vi "Configure Channels.vi"(8 "error in":errorcluster, 11 "AI Voltage DAQmx Cont CFG in":refnum<class "AI Voltage DAQmx Cont CFG.lvclass">) -> (0 "error out":errorcluster, 3 "AI Voltage DAQmx Cont CFG out":refnum<class "AI Voltage DAQmx Cont CFG.lvclass">)   [LabVIEW 2023, in "AI Voltage DAQmx Cont CFG.lvclass"]
uses:
  AI Voltage DAQmx Cont CFG.lvclass
  AI Voltage DAQmx Cont CFG.lvclass/AI Voltage DAQmx Cont CFG.ctl
  <vilib>/Utility/error.llb/Error Cluster From Error Code.vi
  <vilib>/ErrorRing/Error Ring.xnode
  Configuration/Configuration JSON/Configuration JSON Base/CFG JSON.lvclass
  809d0f84-c2e6-4280-b3a5-eb032ce861ff.vi
  DAQmx/DAQmx Base CFG/DAQmx Base CFG.lvclass
  D:/git/HAL/HAL GOOP4/DAQmx/DAQmx BufferLastReadsDBL/DAQmx BufferLastReadsDBL.lvclass
  D:/git/HAL/HAL GOOP4/DAQmx/DAQmx Base CFG/DAQmx Base CFG.lvclass
  D:/git/HAL/HAL GOOP4/CFG Target/CFG Target.lvclass
  D:/git/HAL/HAL GOOP4/Configuration/Configuration Semaphore/CFG Semaphore.lvclass
  D:/git/HAL/HAL GOOP4/Configuration/Configuration JSON/Configuration JSON Base/CFG JSON.lvclass
  D:/git/HAL/HAL GOOP4/Interfaces/IConfigure/IConfigure.lvclass
  D:/git/HAL/HAL GOOP4/AI/AI Voltage DAQmx Cont CFG/AI Voltage DAQmx Cont CFG.lvclass
  <vilib>/DAQmx/create/channels.llb/DAQmx Create Channel (AI-Voltage-Basic).vi
  DAQmx/BufferLastReadingsDBL/BufferLastReadsDBL.lvclass
  DAQmx/DAQmx BufferLastReadsDBL/DAQmx BufferLastReadsDBL.lvclass
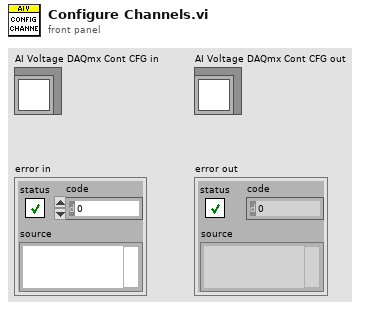
[diagram p1: front panel]
types:
  T1 = cluster{"Name":string, "Enabled":bool, "Max Value":dbl, "Min Value":dbl, "Input Terminal CFG":string, "Units":string, "Shunt Resistor Location":string, "External Shunt Resistor Value":dbl}[]
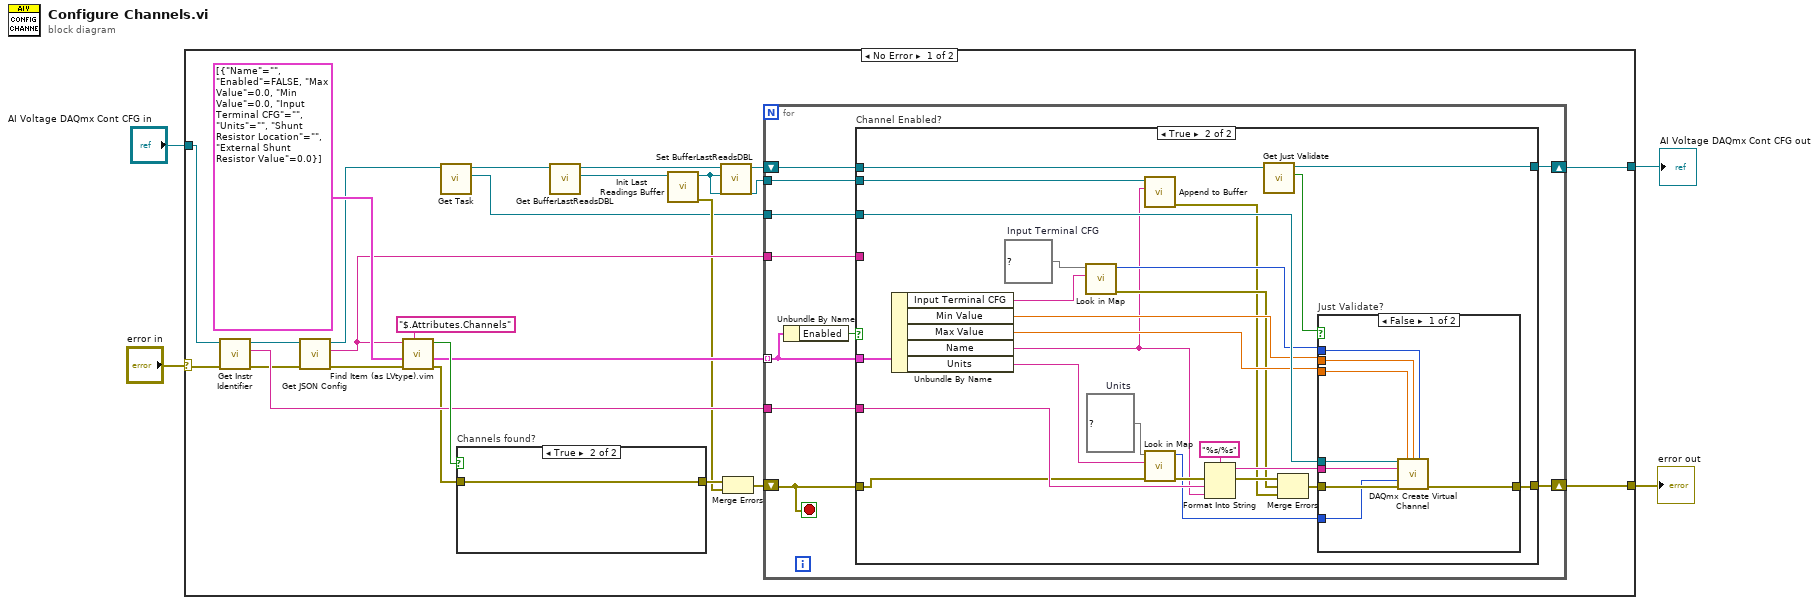
[diagram p0: block diagram]
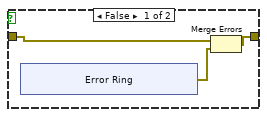
[diagram p2: hidden frame]
diagram:
  n1 = case shown="No Error" "error in" {
    selector: "error in" -> [w21 w83]
    tunnel: "AI Voltage DAQmx Cont CFG in" -> [w18 w84]
    tunnel: [w22 w83] -> w1
    tunnel: [w17 w84] -> w2
    frame No Error {
      n2 = call-dynamic "Get Instr Identifier.vi"("error in"=w21, "Configuration Base in"=w18) -> ("error out"=w14:errorcluster, "Instr Ident"=w23:string, "Configuration Base out"=w24:refnum<class "AI Voltage DAQmx Cont CFG.lvclass">)  [unwired: 7 in]
      n3 = call "Get JSON Config.vi"("CFG Base in"=w24) -> ("<JSON>Config>"=w20:string, "CFG Base out"=w13:refnum<class "AI Voltage DAQmx Cont CFG.lvclass">)  [unwired: 9 in]
      n4 = call "Find Item (as LVtype).vim"("$Path or Item Name"="$.Attributes.Channels", "error in (no error)"=w14, "Data Type and Default Value"=T1 [{"Name"="", "Enabled"=FALSE, "Max Value"=0.0, "Min Value"=0.0, "Input Terminal CFG"="", "Units"="", "Shunt Resistor Location"="", "External Shunt Resistor Value"=0.0}], "JSON"=w20) -> ("error out"=w15:errorcluster, "Data"=w19:T1, "Found"=w26:bool)  [unwired: 4 in, 1 out]
      n5 = call "Get Task.vi"("DAQmx Base CFG in"=w13) -> ("Task"=w10:refnum<k21>, "DAQmx Base CFG out"=w7:refnum<class "AI Voltage DAQmx Cont CFG.lvclass">)  [unwired: 9 in]
      n6 = case "Channels found?" shown="True" w26 {
        tunnel: w15 -> [w30 w36]
        tunnel: [w28 w36] -> w16
        frame False {
          n7 = xnode "Error Ring"() -> ("error out"=w29:errorcluster)
          n8 = Merge Errors(w30, w29) -> (w28:errorcluster)
        }
        frame True {
        }
      }
      n9 = call "Get BufferLastReadsDBL.vi"("DAQmx BufferLastReadsDBL in"=w7) -> ("BufferLastReadsDBL.lvclass"=w5:refnum<class "BufferLastReadsDBL.lvclass">, "DAQmx BufferLastReadsDBL out"=w6:refnum<class "AI Voltage DAQmx Cont CFG.lvclass">)  [unwired: 9 in]
      n10 = call-dynamic "Init Last Readings Buffer.vi"("BufferLastReadingsDBL in"=w5) -> ("error out"=w11:errorcluster, "BufferLastReadingsDBL out"=w8:refnum<class "BufferLastReadsDBL.lvclass">)  [unwired: 9 in]
      n11 = call "Set BufferLastReadsDBL.vi"("BufferLastReadsDBL.lvclass"=w8, "DAQmx BufferLastReadsDBL in"=w6) -> ("DAQmx BufferLastReadsDBL out"=w9:refnum<class "AI Voltage DAQmx Cont CFG.lvclass">)  [unwired: 9 in]
      n12 = Merge Errors(w16, w11) -> (w12:errorcluster)
      n13 = for {
        tunnel: w19 -> [w43] mode=indexing
        shift-right: [w46] -> w22
        shift-left: w12 -> [w45]
        tunnel: w23 -> [w44]
        tunnel: w20 -> [w42]
        tunnel: w10 -> [w41]
        shift-right: [w40] -> w17
        shift-left: w9 -> [w39]
        tunnel: w8 -> [w37]
        stop <- w45 stop-if-true
        n14 = Unbundle By Name(w43) -> ("Enabled"=w38:bool)
        n15 = case "Channel Enabled?" shown="True" w38 {
          tunnel: [w48 w72] -> w46
          tunnel: w45 -> [w48 w54]
          tunnel: w44 -> [_ w66]
          tunnel: w43 -> [_ w73]
          tunnel: [w47 w69] -> w40
          tunnel: w42 -> [_ _]
          tunnel: w41 -> [_ w71]
          tunnel: w39 -> [w47 w70]
          tunnel: w37 -> [_ w53]
          frame False {
          }
          frame True {
            w49 = map{string, i32} {"Default"=-1, "Differential"=10106, "NRSE"=10078, "Pseudodifferential"=12529, "RSE"=10083}  # Input Terminal CFG
            w50 = map{string, i32} {"From Custom Scale"=10065, "Volts"=10348}  # Units
            n16 = Unbundle By Name(w73) -> ("Input Terminal CFG"=w62:string, "Min Value"=w60:dbl, "Max Value"=w59:dbl, "Name"=w52:string, "Units"=w57:string)
            n17 = call "Look in Map.vi"("Key"=w62, "Map"=w49) -> ("error out"=w56:errorcluster, "Value"=w61:i32)  [unwired: 8 in]
            n18 = call-dynamic "Append to Buffer.vi"("Channel"=w52, "BufferLastReadingsDBL in"=w53) -> ("error out"=w51:errorcluster)  [unwired: 8 in, 1 out]
            n19 = call "Look in Map.vi"("error in"=w54, "Key"=w57, "Map"=w50) -> ("error out"=w58:errorcluster, "Value"=w55:i32)  [unwired: 7 in]
            n20 = Format Into String(format string="%s/%s", error in=w58, w66, w52) -> (resulting string=w64:string, error out=w65:errorcluster)  [unwired: 1 in]
            n21 = call "Get Just Validate.vi"("CFG JSON Base in"=w70) -> ("Just Validate"=w68:bool, "CFG JSON Base out"=w69:refnum<class "AI Voltage DAQmx Cont CFG.lvclass">)  [unwired: 9 in]
            n22 = Merge Errors(w65, w56, w51) -> (w63:errorcluster)
            n23 = case "Just Validate?" shown="False" w68 {
              tunnel: w63 -> [w81 w82]
              tunnel: w64 -> [w78 _]
              tunnel: w71 -> [w80 _]
              tunnel: [w79 w82] -> w72
              tunnel: w61 -> [w74 _]
              tunnel: w60 -> [w77 _]
              tunnel: w59 -> [w76 _]
              tunnel: w55 -> [w75 _]
              frame False {
                n24 = call-poly <vilib>:"DAQmx Create Virtual Channel.vi"("task in"=w80, "maximum value"=w76, "minimum value"=w77, "input terminal configuration"=w74, "physical channels"=w78, "units"=w75, "error in"=w81) -> ("error out"=w79:errorcluster)  [unwired: 7 in, 1 out]
              }
              frame True {
              }
            }
          }
        }
      }
    }
    frame Error {
    }
  }
  "error out" <- w1
  "AI Voltage DAQmx Cont CFG out" <- w2
